vi "HAL Shutdown.vi"(8 "error in (no error)":errorcluster, 11 "HAL Interface Actor in":refnum<class "HAL Interface Actor.lvclass">) -> (0 "error out":errorcluster, 3 "HAL Interface Actor out":refnum<class "HAL Interface Actor.lvclass">)   [LabVIEW 2024, in "HAL Interface Actor.lvlib" / "HAL Interface Actor.lvclass"]
uses:
  HAL Interface Actor.lvclass
  HAL Interface Actor.lvclass/HAL Interface Actor.ctl
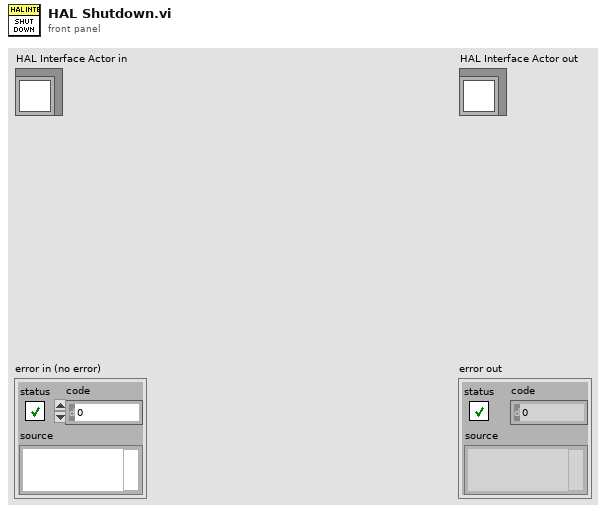
[diagram p1: front panel]
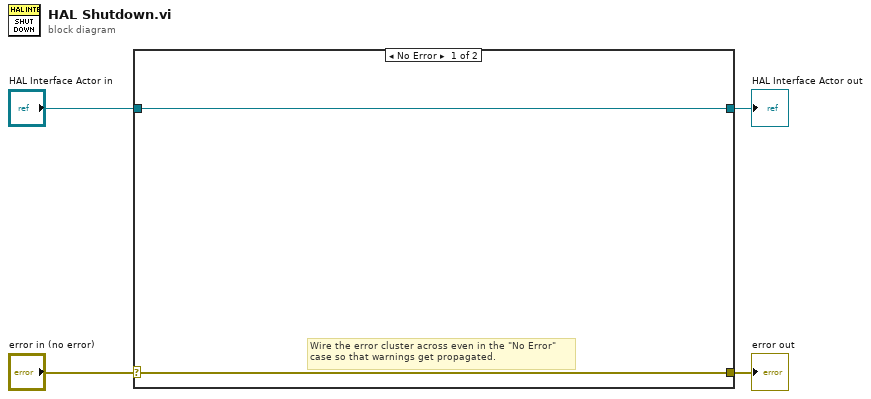
[diagram p0: block diagram]
diagram:
  n1 = case shown="No Error" "error in (no error)" {
    selector: "error in (no error)" -> [w5 w8]
    tunnel: [w5 w8] -> w3
    tunnel: [w6 w7] -> w1
    tunnel: "HAL Interface Actor in" -> [w6 w7]
    frame No Error {
      # "Wire the error cluster across even in the \"No Error\"\ncase so that warnings get propagated."
    }
    frame Error {
    }
  }
  "error out" <- w3
  "HAL Interface Actor out" <- w1
